vi "get_subcomponents.vi"(8 "error in (no error)":errorcluster, 11 "GenericComponent in":refnum<class "GenericComponent.lvclass">) -> (0 "error out":errorcluster, 2 "subcomponents":T1[](array[typedef]), 3 "GenericComponent out":refnum<class "GenericComponent.lvclass">)   [LabVIEW 2010, in "GenericComponent.lvclass"]
uses:
  GenericComponent.lvclass
  subcomponent_cluster.ctl
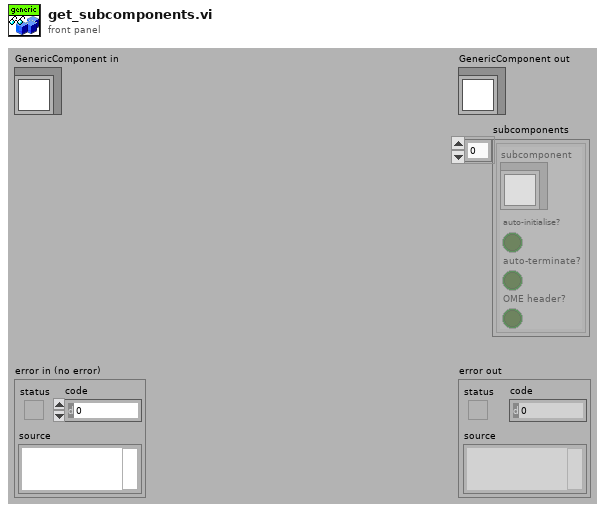
[diagram p1: front panel]
types:
  T1 = typedef "subcomponent_cluster.ctl" = cluster{"subcomponent":refnum<class "GenericComponent.lvclass">, "auto-initialise?":bool, "auto-terminate?":bool, "OME header?":bool}
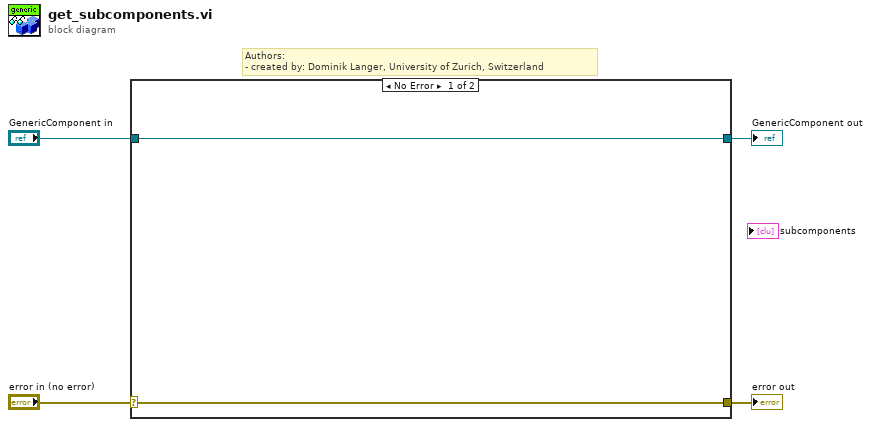
[diagram p0: block diagram]
diagram:
  # "Authors: \n- created by: Dominik Langer, University of Zurich, Switzerland"
  n1 = case shown="No Error" "error in (no error)" {
    selector: "error in (no error)" -> [w5 w8]
    tunnel: [w5 w8] -> w3
    tunnel: [w6 w7] -> w1
    tunnel: "GenericComponent in" -> [w6 w7]
    frame No Error {
    }
    frame Error {
    }
  }
  "error out" <- w3
  "GenericComponent out" <- w1
